vi "Read From Stream.vi"(5 "Upload Path (Temp)":path=path "", 6 "Max Size (50MB)":u64=52428800, 7 "Uploads as Files? (T)":bool=TRUE, 8 "error in (no error)":errorcluster, 9 "TCP in":refnum<k5>, 10 "Client URI":refnum<class "URI.lvclass">) -> (0 "error out":errorcluster, 1 "TCP":refnum<k5>, 3 "Request out":refnum<class "Request.lvclass">)   [LabVIEW 2020, in "HTTP Utils.lvlib" / "Request.lvclass"]
uses:
  Request.lvclass
  Request.lvclass/Request.ctl
  HTTP Utils.lvlib
  lv-uri/URI/URI/URI.lvclass
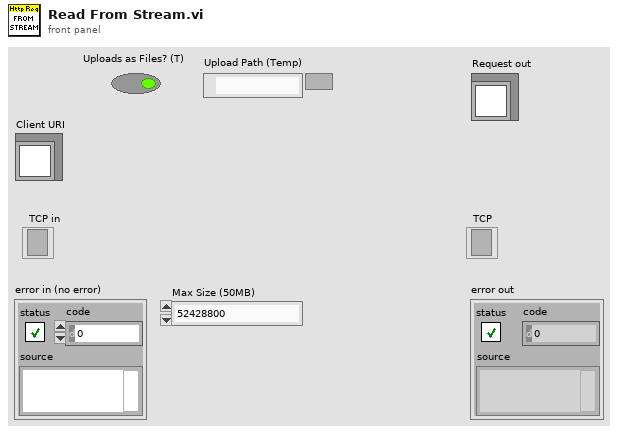
[diagram p1: front panel]
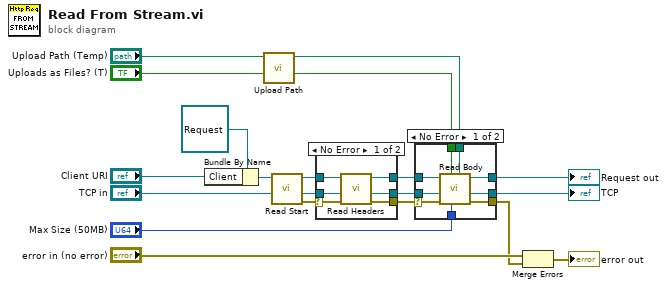
[diagram p0: block diagram]
diagram:
  n1 = Bundle By Name(cluster=refnum<class "Request.lvclass"> refnum ("Request in"), "Client"="Client URI") -> (w15:refnum<class "Request.lvclass">)
  n2 = call "Upload Path.vi"("Specified Path (Temp)"="Upload Path (Temp)") -> ("Upload Path"=w12:path)  [unwired: 10 in]
  n3 = call "Read Start.vi"("Stream in"="TCP in", "Request in"=w15) -> ("error out"=w8:errorcluster, "Stream out"=w7:refnum<k5>, "Request out"=w9:refnum<class "Request.lvclass">)  [unwired: 7 in]
  n4 = case shown="No Error" w8 {
    selector: w8 -> [w23 w28]
    tunnel: [w25 w28] -> w10
    tunnel: w9 -> [w24 w26]
    tunnel: w7 -> [w22 w27]
    tunnel: [w21 w26] -> w6
    tunnel: [w20 w27] -> w5
    frame No Error {
      n5 = call "Read Headers.vi"("error in (no error)"=w23, "Stream in"=w22, "Request in"=w24) -> ("error out"=w25:errorcluster, "Stream out"=w20:refnum<k5>, "Request out"=w21:refnum<class "Request.lvclass">)  [unwired: 5 in, 1 out]
    }
    frame Error {
    }
  }
  n6 = case shown="No Error" w10 {
    selector: w10 -> [w37 w38]
    tunnel: w6 -> [w36 w40]
    tunnel: w5 -> [w35 w39]
    tunnel: [w34 w40] -> w16
    tunnel: [w33 w39] -> w1
    tunnel: [w32 w38] -> w4
    tunnel: "Uploads as Files? (T)" -> [w31 _]
    tunnel: w12 -> [w30 _]
    tunnel: "Max Size (50MB)" -> [w29 _]
    frame No Error {
      n7 = call "Read Body.vi"("Upload Path"=w30, "Max Size (50MB)"=w29, "Uploads as Files? (T)"=w31, "error in (no error)"=w37, "Stream in"=w35, "Request in"=w36) -> ("error out"=w32:errorcluster, "Stream out"=w33:refnum<k5>, "Request out"=w34:refnum<class "Request.lvclass">)  [unwired: 3 in]
    }
    frame Error {
    }
  }
  "Request out" <- w16
  "TCP" <- w1
  n8 = Merge Errors("error in (no error)", w4) -> (→"error out":errorcluster)
